vi "ATA10003-Read.vi"(1 "Address(0x01)":u8=1 format="%.0x", 7 "Function_In":string(combo)="ReadVrms", 11 "error in":errorcluster) -> (6 "Measured":dbl, 15 "error out":errorcluster)   [LabVIEW 2015]
uses:
  <vilib>/Instr/_visa.llb/VISA Configure Serial Port (Instr).vi
panel:
  out "VISA":refnum<visa-resource-name>
  in  "MyIndex":u8
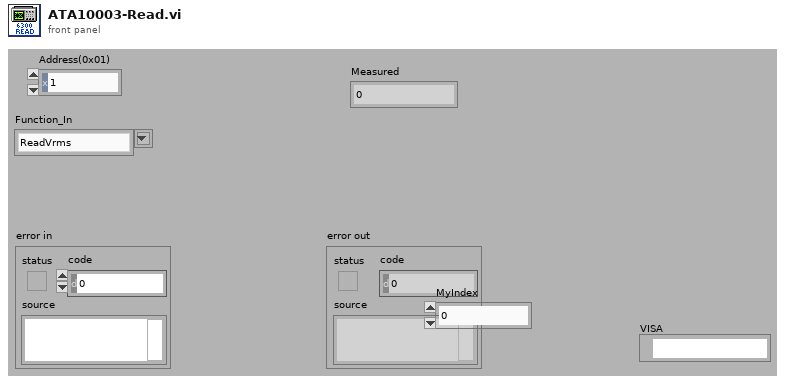
[diagram p1: front panel]
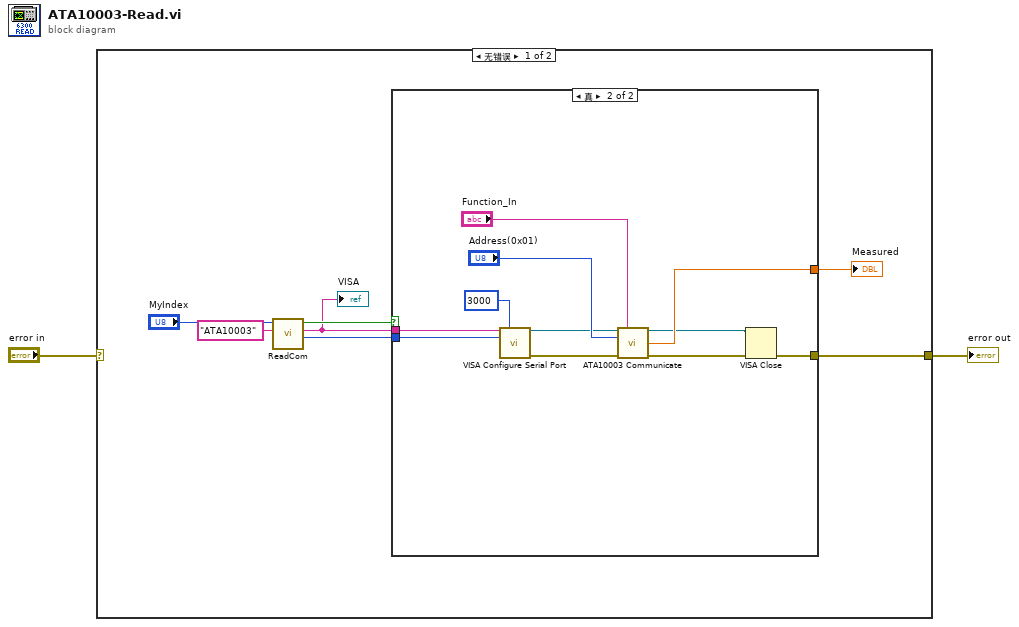
[diagram p0: block diagram]
diagram:
  n1 = case shown="无错误" "error in" {
    selector: "error in" -> [_ w21]
    tunnel: [w8 w21] -> w2
    frame No Error {
      n2 = call "ReadCom.vi"("仪器名称"="ATA10003", "MyIndex"="MyIndex") -> ("Baudrate"=w3:i32, "COM"=w4:string, "OK?"=w5:bool)  [unwired: 7 in]
      "VISA" <- w4
      n3 = case shown="真" w5 {
        tunnel: [_ w18] -> w9
        tunnel: [_ w16] -> w8
        tunnel: w4 -> [_ w12]
        tunnel: w3 -> [_ w11]
        frame False {
        }
        frame True {
          n4 = call-poly "VISA Configure Serial Port"("VISA resource name"=w12, "timeout (10sec)"=u32 3000, "baud rate (9600)"=w11) -> ("VISA resource name out"=w13:refnum<visa-resource-name>, "error out"=w14:errorcluster)  [unwired: 11 in]
          n5 = call "ATA10003 Communicate.vi"("VISA Resource In"=w13, "Function_In"="Function_In", "Address(0x01)"="Address(0x01)", "error in (no error)"=w14) -> ("VISA Resource Out"=w15:refnum<visa-resource-name>, "Value"=w18:dbl, "error out"=w17:errorcluster)  [unwired: 7 in, 2 out]
          n6 = VISA Close(VISA resource name=w15, error in (no error)=w17) -> (error out=w16:errorcluster)
        }
      }
      "Measured" <- w9
    }
    frame Error {
    }
  }
  "error out" <- w2
